vi "calc_SolutionChangeWaveform_v0.03.vi"(0 "New input cluster":T1={"Which Position to use for Experiment"=enum."Jumper Safe Position", "Duration (s)"=60.0, "Delay (s)"=1.0, "Pulse Width (s)"=30.0, "Which Valve to Change?"=1, "Valve Jump Position"=3, "Replicates"=1.0, "Vholding (mV)"=-70.0, "valve 1 used now?"=TRUE, "valve 2 used now?"=FALSE, "valve 3 used now? "=FALSE, "Valve 1 Position"=2, "Valve 2 Position"=2, "Valve 3 Position"=2, "protocol Preview"=[]} {"Valve 3 Position" min=1 max=8; "Valve 2 Position" min=1 max=8; "Valve 1 Position" min=1 max=8; "Delay (s)" min=0.0 step=0.1; "Duration (s)" min=0.0 step=0.1}, 1 "Clear Waveform?":bool, 5 "Old input cluster":T1={"Which Position to use for Experiment"=enum."Jumper Safe Position", "Duration (s)"=60.0, "Delay (s)"=1.0, "Pulse Width (s)"=30.0, "Which Valve to Change?"=1, "Valve Jump Position"=3, "Replicates"=1.0, "Vholding (mV)"=-70.0, "valve 1 used now?"=TRUE, "valve 2 used now?"=FALSE, "valve 3 used now? "=FALSE, "Valve 1 Position"=2, "Valve 2 Position"=2, "Valve 3 Position"=2, "protocol Preview"=[]} {"Valve 3 Position" min=1 max=8; "Valve 2 Position" min=1 max=8; "Valve 1 Position" min=1 max=8; "Delay (s)" min=0.0 step=0.1; "Duration (s)" min=0.0 step=0.1}, 7 "sample freq":i32=10000, 11 "error in":errorcluster) -> (4 "output cluster":T1={"Which Position to use for Experiment"=enum."Jumper Safe Position", "Duration (s)"=60.0, "Delay (s)"=1.0, "Pulse Width (s)"=30.0, "Which Valve to Change?"=1, "Valve Jump Position"=3, "Replicates"=1.0, "Vholding (mV)"=-70.0, "valve 1 used now?"=TRUE, "valve 2 used now?"=FALSE, "valve 3 used now? "=FALSE, "Valve 1 Position"=2, "Valve 2 Position"=2, "Valve 3 Position"=2, "protocol Preview"=[]} {"Valve 3 Position" min=1 max=8; "Valve 2 Position" min=1 max=8; "Valve 1 Position" min=1 max=8; "Delay (s)" min=0.0 step=0.1; "Duration (s)" min=0.0 step=0.1}, 15 "error out":errorcluster)   [LabVIEW 2019]
uses:
  <vilib>/measure/NI_MABase.lvlib
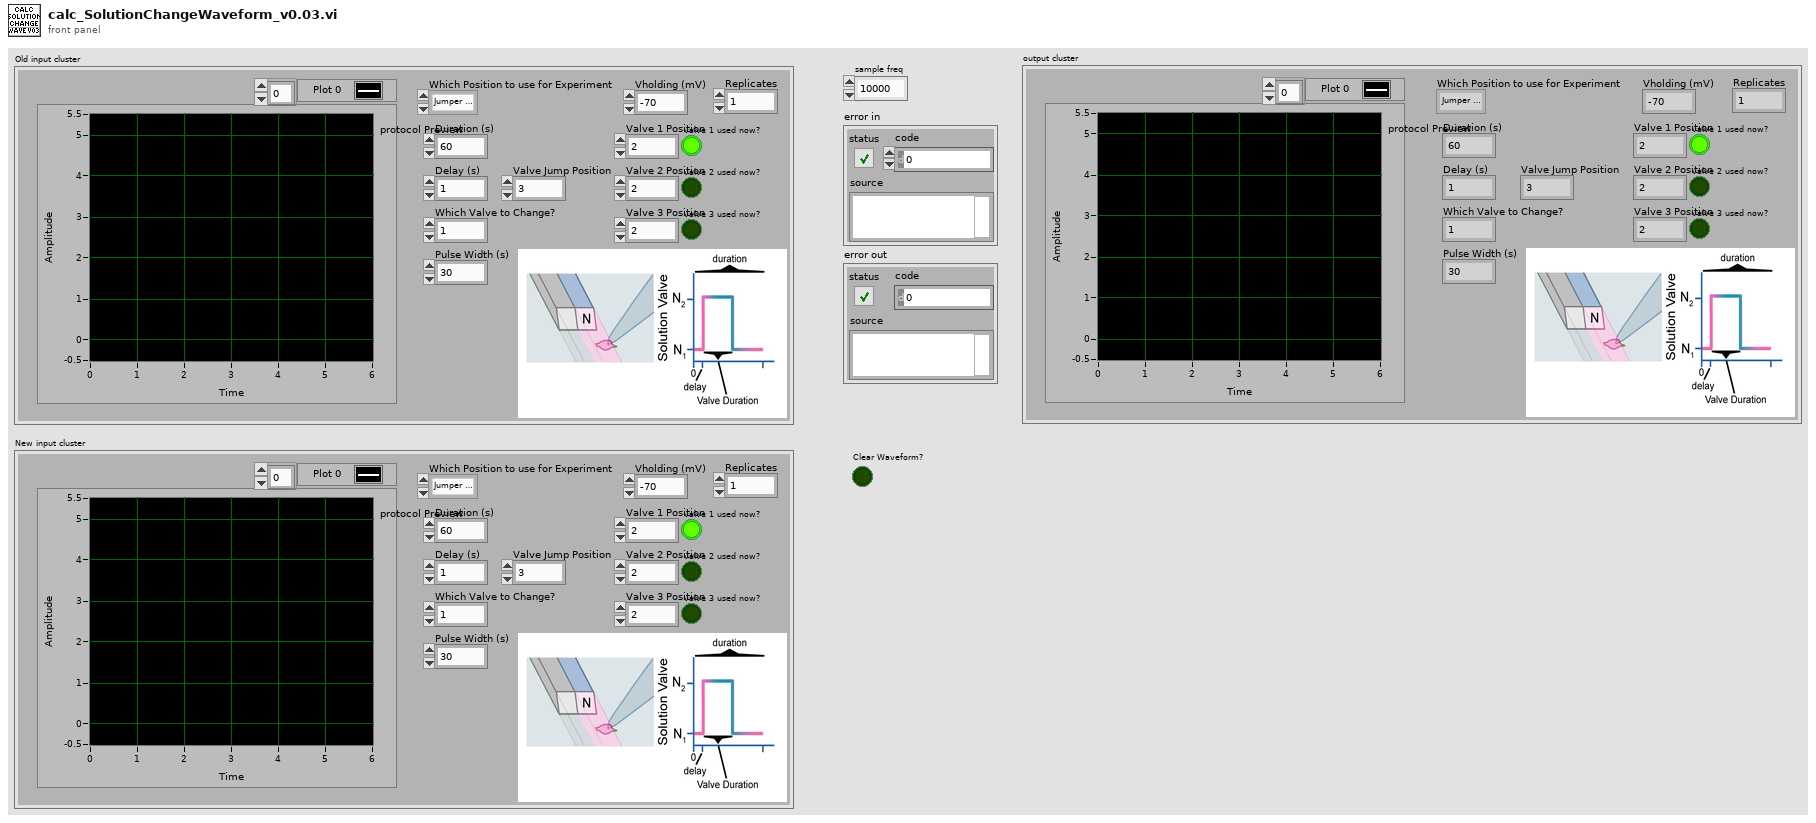
[diagram p1: front panel]
types:
  T1 = cluster{"Which Position to use for Experiment":enum16{"Jumper Safe Position", "Experiment Safe Position", "Jumper Position A", "Jumper Position B", "Jumper Position C", "Jumper Position o-A", "Jumper Position A-o", "Jumper Position A-B", "Jumper Position B-A", "Jumper Position B-C", "Jumper Position C-B", "Jumper Position C-o", "Jumper Position o-C", "Don't Move"}, "Duration (s)":dbl, "Delay (s)":dbl, "Pulse Width (s)":dbl, "Which Valve to Change?":i16, "Valve Jump Position":i16, "Replicates":dbl, "Vholding (mV)":dbl, "valve 1 used now?":bool, "valve 2 used now?":bool, "valve 3 used now? ":bool, "Valve 1 Position":i16, "Valve 2 Position":i16, "Valve 3 Position":i16, "protocol Preview":waveform(dbl)[]}
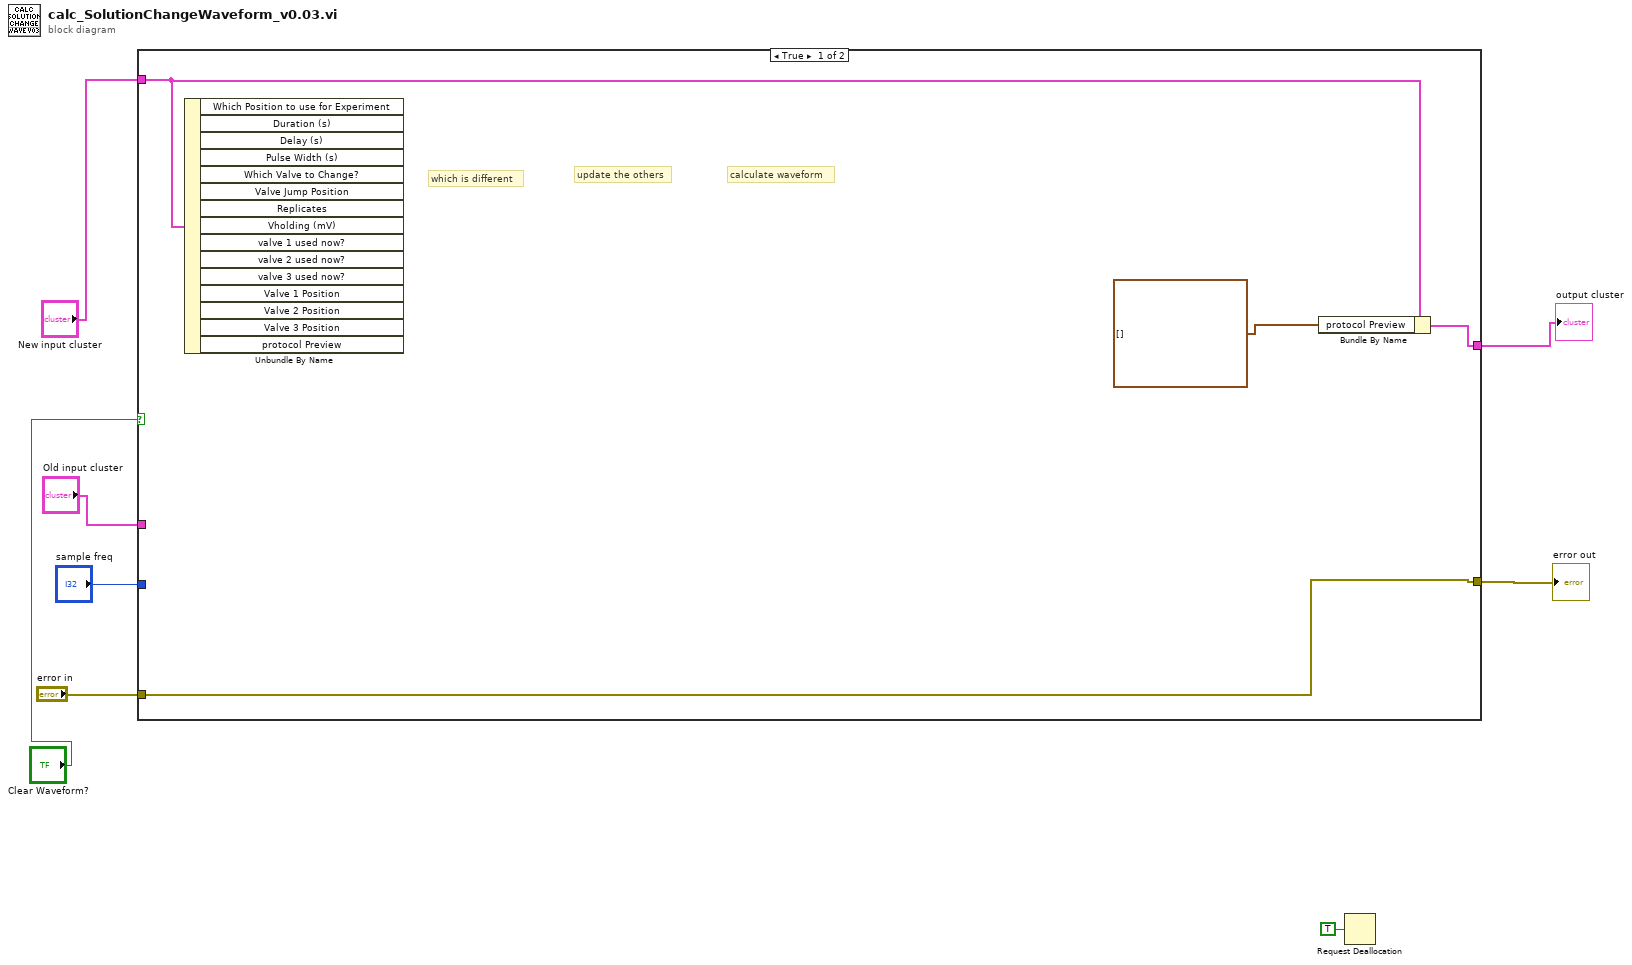
[diagram p0: block diagram]
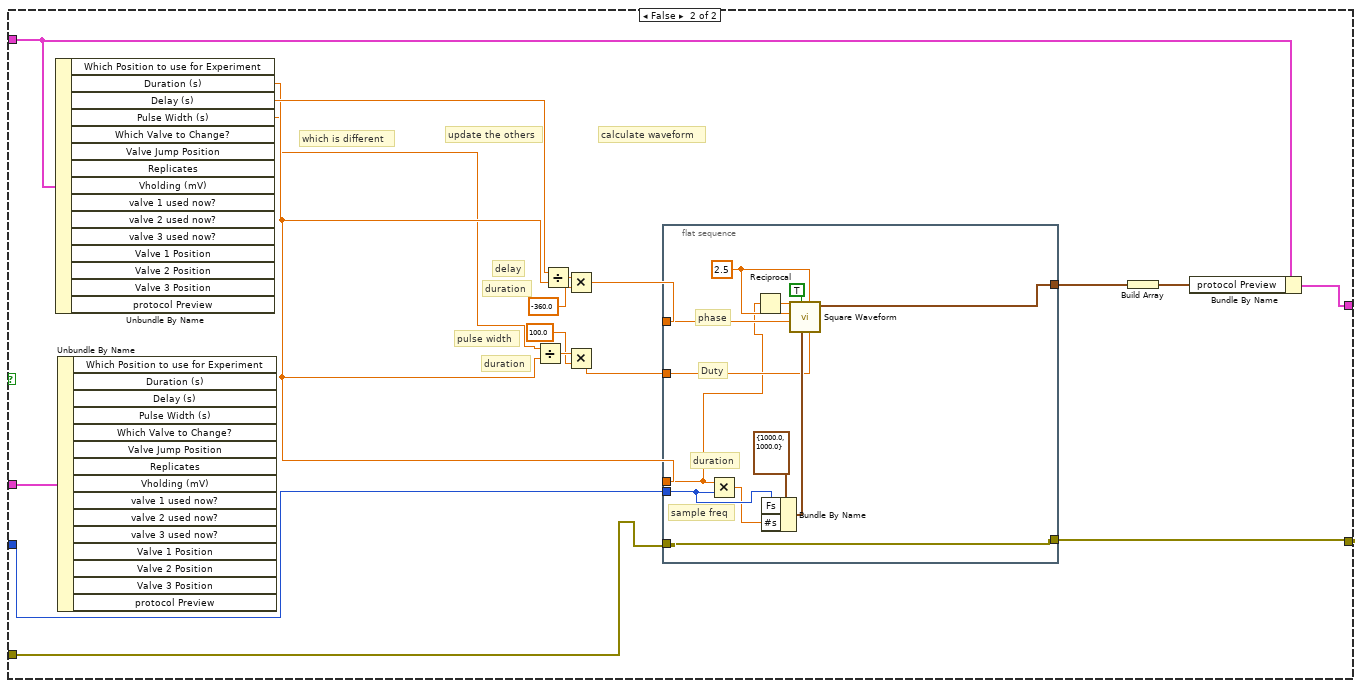
[diagram p2: hidden frame]
diagram:
  n1 = case shown="True" "Clear Waveform?" {
    tunnel: "New input cluster" -> [w12 w29]
    tunnel: [w11 w28] -> w7
    tunnel: "Old input cluster" -> [_ w27]
    tunnel: "sample freq" -> [_ w25]
    tunnel: "error in" -> [w9 w24]
    tunnel: [w9 w19] -> w3
    frame True {
      # "calculate waveform"
      # "update the others"
      # "which is different"
      n2 = Unbundle By Name(w12) -> ()  [unwired: 15 out]
      n3 = Bundle By Name(cluster=w12, "protocol Preview"=waveform(dbl)[] []) -> (w11:T1)
    }
    frame False {
      # "pulse width"
      # "duration"
      # "duration"
      # "delay"
      # "calculate waveform"
      # "update the others"
      # "which is different"
      n4 = Unbundle By Name(w29) -> ("Duration (s)"=w22:dbl, "Delay (s)"=w23:dbl, "Pulse Width (s)"=w21:dbl)  [unwired: 12 out]
      n5 = Unbundle By Name(w27) -> ()  [unwired: 15 out]
      n6 = Divide(x=w21, y=w22) -> (x/y=w16:dbl)
      n7 = Divide(x=w23, y=w22) -> (x/y=w18:dbl)
      n8 = Multiply(x=w18, y=-360.0) -> (x*y=w14:dbl)
      n9 = Multiply(x=w16, y=100.0) -> (x*y=w13:dbl)
      n10 = flat-sequence {
        tunnel: w14 -> [w36]
        tunnel: w13 -> [w37]
        tunnel: w22 -> [w33]
        tunnel: w24 -> [w31]
        tunnel: w25 -> [w34]
        tunnel: [w32] -> w20
        tunnel: [w31] -> w19
        frame #0 {
          w41 = 2.5 ("Amplitude")
          # "sample freq"
          # "duration"
          # "Duty"
          # "phase"
          n11 = Multiply(x=w33, y=w34) -> (x*y=w30:dbl)
          n12 = Reciprocal(x=w33) -> (1/x=w35:dbl)
          n13 = Bundle By Name(cluster=cluster{"Fs":dbl, "#s":dbl} {"Fs"=1000.0, "#s"=1000.0} ("sampling info"), "Fs"=w34, "#s"=w30) -> (w38:cluster{"Fs":dbl, "#s":dbl})
          n14 = call <vilib>:"Square Waveform.vi"("duty cycle (%)"=w37, "offset"=w41, "sampling info"=w38, "reset signal"=TRUE, "phase"=w36, "amplitude"=w41, "frequency"=w35) -> ("signal out"=w32:waveform(dbl))  [unwired: 3 in, 1 out]
        }
      }
      n15 = Build Array(w20) -> (w26:waveform(dbl)[])
      n16 = Bundle By Name(cluster=w29, "protocol Preview"=w26) -> (w28:T1)
    }
  }
  "output cluster" <- w7
  "error out" <- w3
  n17 = Request Deallocation(TRUE ("flag")) -> ()
